vi "Asylum_SetInWave.vi"(4 "decimation":i32, 6 "callback":string, 7 "whichBank":i32, 8 "error in (no error)":errorcluster, 9 "Wave":cluster{"channelString":string, "wave":string}, 10 "eventString":string, 11 "Application":refnum<k7>) -> (0 "error out":errorcluster, 3 "Application":refnum<k7>)   [LabVIEW 2020]
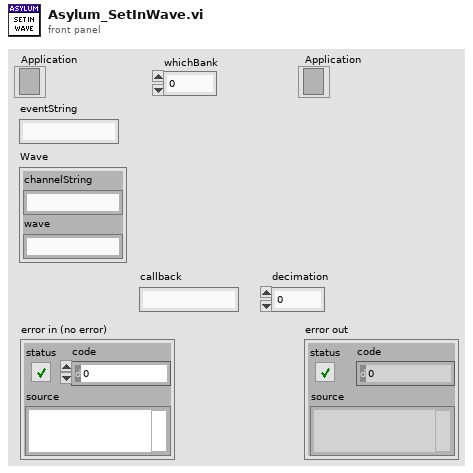
[diagram p1: front panel]
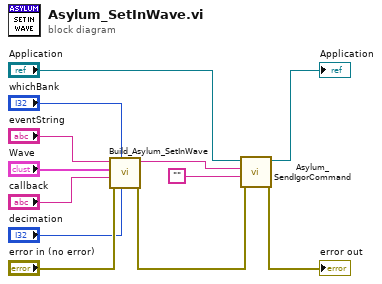
[diagram p0: block diagram]
diagram:
  n1 = call "Build_Asylum_SetInWave.vi"("decimation"="decimation", "whichBank"="whichBank", "error in (no error)"="error in (no error)", "callback"="callback", "Wave"="Wave", "eventString"="eventString") -> ("error out"=w12:errorcluster, "Command"=w10:string)  [unwired: 4 in]
  n2 = call "Asylum_SendIgorCommand.vi"("error in (no error)"=w12, "Format"="", "command"=w10, "Application"="Application") -> ("error out"=→"error out":errorcluster, "Application"=→"Application":refnum<k7>)  [unwired: 4 in, 2 out]
